vi "loadClassLabels.vi"(8 "error in (no error)":errorcluster, 10 "dict path":path, 11 "dl in":refnum<class "dl.lvclass">) -> (0 "error out":errorcluster, 2 "loadSucc":i32, 3 "dl out":refnum<class "dl.lvclass">)   [LabVIEW 2025, in "dl.lvlib" / "dl.lvclass"]
uses:
  dl.lvclass
  dl.lvclass/dl.ctl
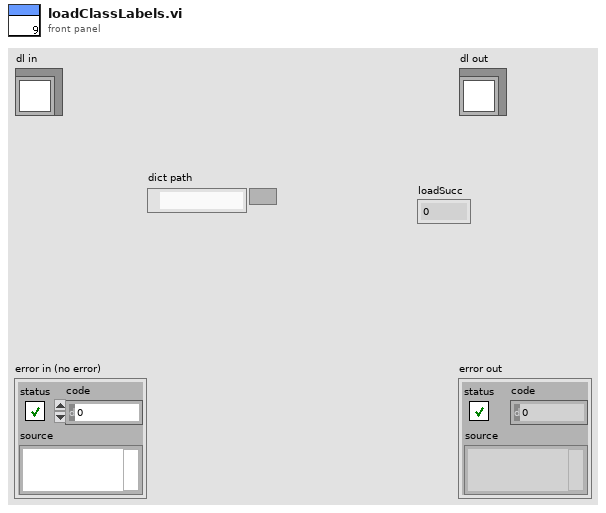
[diagram p1: front panel]
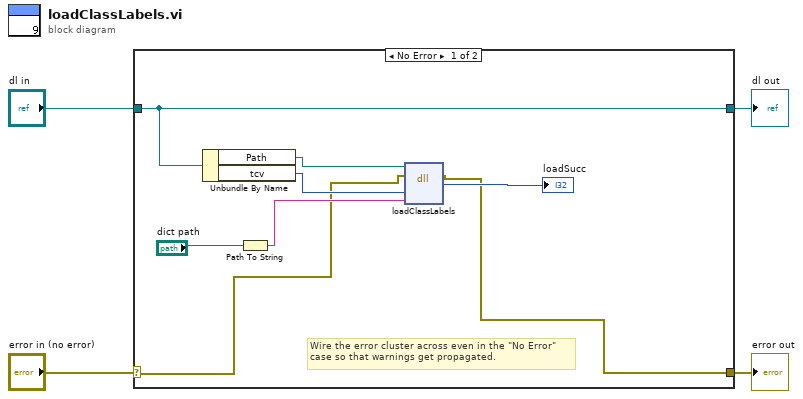
[diagram p0: block diagram]
diagram:
  n1 = case shown="No Error" "error in (no error)" {
    selector: "error in (no error)" -> [w6 w14]
    tunnel: [w5 w14] -> w3
    tunnel: [w12 w13] -> w1
    tunnel: "dl in" -> [w12 w13]
    frame No Error {
      # "Wire the error cluster across even in the \"No Error\"\ncase so that warnings get propagated."
      n2 = Unbundle By Name(w12) -> ("Path"=w11:path, "tcv"=w10:u64)
      n3 = Path To String(path="dict path") -> (string=w7:string)
      n4 = dll-call lib="D:/Test/adslvPackageDev/Resources/TCV_Lib.dll" fn="loadClassLabels"(path in=w11, error in=w6, "tcv"=w10, "dictpath"=w7) -> (error out=w5:errorcluster, "loadSucc"=→"loadSucc":i32)  [unwired: 3 in, 1 out]
    }
    frame Error {
    }
  }
  "error out" <- w3
  "dl out" <- w1
